vi "System8.vi"() -> ()   [LabVIEW 2015]
uses:
  Control 1.ctl
  <vilib>/DAQmx/write.llb/DAQmx Write (Digital 1D Bool NChan 1Samp 1Line).vi
  <vilib>/DAQmx/write.llb/DAQmx Write (Digital Bool 1Line 1Point).vi
  <vilib>/DAQmx/read.llb/DAQmx Read (Analog DBL 1Chan 1Samp).vi
  <vilib>/DAQmx/read.llb/DAQmx Read (Analog 1D Wfm NChan NSamp).vi
  <vilib>/Analysis/baseanly.llb/Mean (DBL).vi
  <vilib>/DAQmx/write.llb/DAQmx Write (Analog DBL 1Chan 1Samp).vi
  <vilib>/DAQmx/miscellaneous.llb/DAQmx Fill In Error Info.vi
  <vilib>/addons/control/pid/NI_PID_autopid.lvlib
  <vilib>/Analysis/NI_AALBase.lvlib
panel:
  out "Voltage Reading(Temp) 2":dbl format="%#_13g"
  out "Temperature (Celcius) 2":dbl format="%#.1g"
  out "Temp(C) 2":dbl(slide) scale=-10.0..100.0
  out "Temp Chart 3":waveform(dbl)(graph)
  in  "autotuning parameters 4":T1={"controller type"=1, "relay cycles"=3, "relay amplitude"=1.0, "control specification"=2, "PV noise level"=0.1} {"PV noise level" format="%.2f"; "control specification" items=["normal", "fast", "slow"]; "relay amplitude" format="%.2f"; "controller type" items=["PID", "PI", "P"]}
  in  "PID gains 4":T2={"proportional gain (Kc)"=1.0, "integral time (Ti, min)"=0.01, "derivative time (Td, min)"=0.0} {"derivative time (Td, min)" format="%.3f"; "integral time (Ti, min)" format="%.3f"; "proportional gain (Kc)" format="%.3f"}
  out "PID gains out 4":T2={"proportional gain (Kc)"=1.0, "integral time (Ti, min)"=0.01, "derivative time (Td, min)"=0.0} {"derivative time (Td, min)" format="%.3f"; "integral time (Ti, min)" format="%.3f"; "proportional gain (Kc)" format="%.3f"}
  in  "autotune? (F) 4":bool
  in  "reinitialize? (F) 4":bool
  in  "setpoint in C 2":dbl format="%.2f"
  in  "Manual Control 4":bool
  in  "Heater On/Off 2":bool
  out "Voltage Reading(Temp)":dbl format="%#_13g"
  out "Temperature (Celcius)":dbl format="%#.1g"
  out "Temp(C)":dbl(slide) scale=-10.0..100.0
  out "Temp Chart 2":waveform(dbl)(graph)
  in  "autotuning parameters 3":T1={"controller type"=1, "relay cycles"=3, "relay amplitude"=1.0, "control specification"=2, "PV noise level"=0.1} {"PV noise level" format="%.2f"; "control specification" items=["normal", "fast", "slow"]; "relay amplitude" format="%.2f"; "controller type" items=["PID", "PI", "P"]}
  in  "PID gains 3":T2={"proportional gain (Kc)"=1.0, "integral time (Ti, min)"=0.01, "derivative time (Td, min)"=0.0} {"derivative time (Td, min)" format="%.3f"; "integral time (Ti, min)" format="%.3f"; "proportional gain (Kc)" format="%.3f"}
  out "PID gains out 3":T2={"proportional gain (Kc)"=1.0, "integral time (Ti, min)"=0.01, "derivative time (Td, min)"=0.0} {"derivative time (Td, min)" format="%.3f"; "integral time (Ti, min)" format="%.3f"; "proportional gain (Kc)" format="%.3f"}
  in  "autotune? (F) 3":bool
  in  "reinitialize? (F) 3":bool
  in  "setpoint in C":dbl format="%.2f"
  out "Control Value 3":dbl
  in  "Manual Control 3":bool
  in  "Heater On/Off":bool
  in  "Open/Close (Green)":bool
  in  "Open/Close (Blue)":bool
  in  "Stop program":bool
  in  "On/Off":bool
  in  "Manual Control 2":bool
  in  "Voltage setting 2":dbl format="%#_13g"
  out "Voltage Reading(pressure) 2":dbl format="%#_13g"
  out "Pressure 2":dbl format="%#.3g"
  out "Pressure Chart 2":dbl(graph)
  in  "autotuning parameters 2":T1={"controller type"=1, "relay cycles"=3, "relay amplitude"=1.0, "control specification"=2, "PV noise level"=0.1} {"PV noise level" format="%.2f"; "control specification" items=["normal", "fast", "slow"]; "relay amplitude" format="%.2f"; "controller type" items=["PID", "PI", "P"]}
  in  "PID gains 2":T2={"proportional gain (Kc)"=1.0, "integral time (Ti, min)"=0.01, "derivative time (Td, min)"=0.0} {"derivative time (Td, min)" format="%.3f"; "integral time (Ti, min)" format="%.3f"; "proportional gain (Kc)" format="%.3f"}
  out "PID gains out 2":T2={"proportional gain (Kc)"=1.0, "integral time (Ti, min)"=0.01, "derivative time (Td, min)"=0.0} {"derivative time (Td, min)" format="%.3f"; "integral time (Ti, min)" format="%.3f"; "proportional gain (Kc)" format="%.3f"}
  in  "autotune? (F) 2":bool
  in  "reinitialize? (F) 2":bool
  in  "setpoint in Bar 2":dbl format="%#.5f"
  out "Control Value 2":dbl
  in  "Voltage setting":dbl format="%#_13g"
  in  "Manual Control":bool
  out "Control Value":dbl
  in  "setpoint in Bar":dbl format="%#.5f"
  in  "reinitialize? (F)":bool
  in  "autotune? (F)":bool
  out "PID gains out":T2={"proportional gain (Kc)"=1.0, "integral time (Ti, min)"=0.01, "derivative time (Td, min)"=0.0} {"derivative time (Td, min)" format="%.3f"; "integral time (Ti, min)" format="%.3f"; "proportional gain (Kc)" format="%.3f"}
  in  "PID gains":T2={"proportional gain (Kc)"=1.0, "integral time (Ti, min)"=0.01, "derivative time (Td, min)"=0.0} {"derivative time (Td, min)" format="%.3f"; "integral time (Ti, min)" format="%.3f"; "proportional gain (Kc)" format="%.3f"}
  in  "autotuning parameters":T1={"controller type"=1, "relay cycles"=3, "relay amplitude"=1.0, "control specification"=2, "PV noise level"=0.1} {"PV noise level" format="%.2f"; "control specification" items=["normal", "fast", "slow"]; "relay amplitude" format="%.2f"; "controller type" items=["PID", "PI", "P"]}
  out "Pressure Chart":dbl(graph)
  out "Pressure":dbl format="%#.3g"
  out "Voltage Reading(pressure)":dbl format="%#_13g"
  # "Valves"
  # "Pump 3"
  # "Pressure Vessel 2"
  # "Pressure Vessel 1"
  # "Readings"
  # "Controls"
  # "Readings"
  # "Controls"
  # "PID Settings"
  # "51.12139\n\n0.044676"
  # "Temperature 1"
  # "Temperature 2"
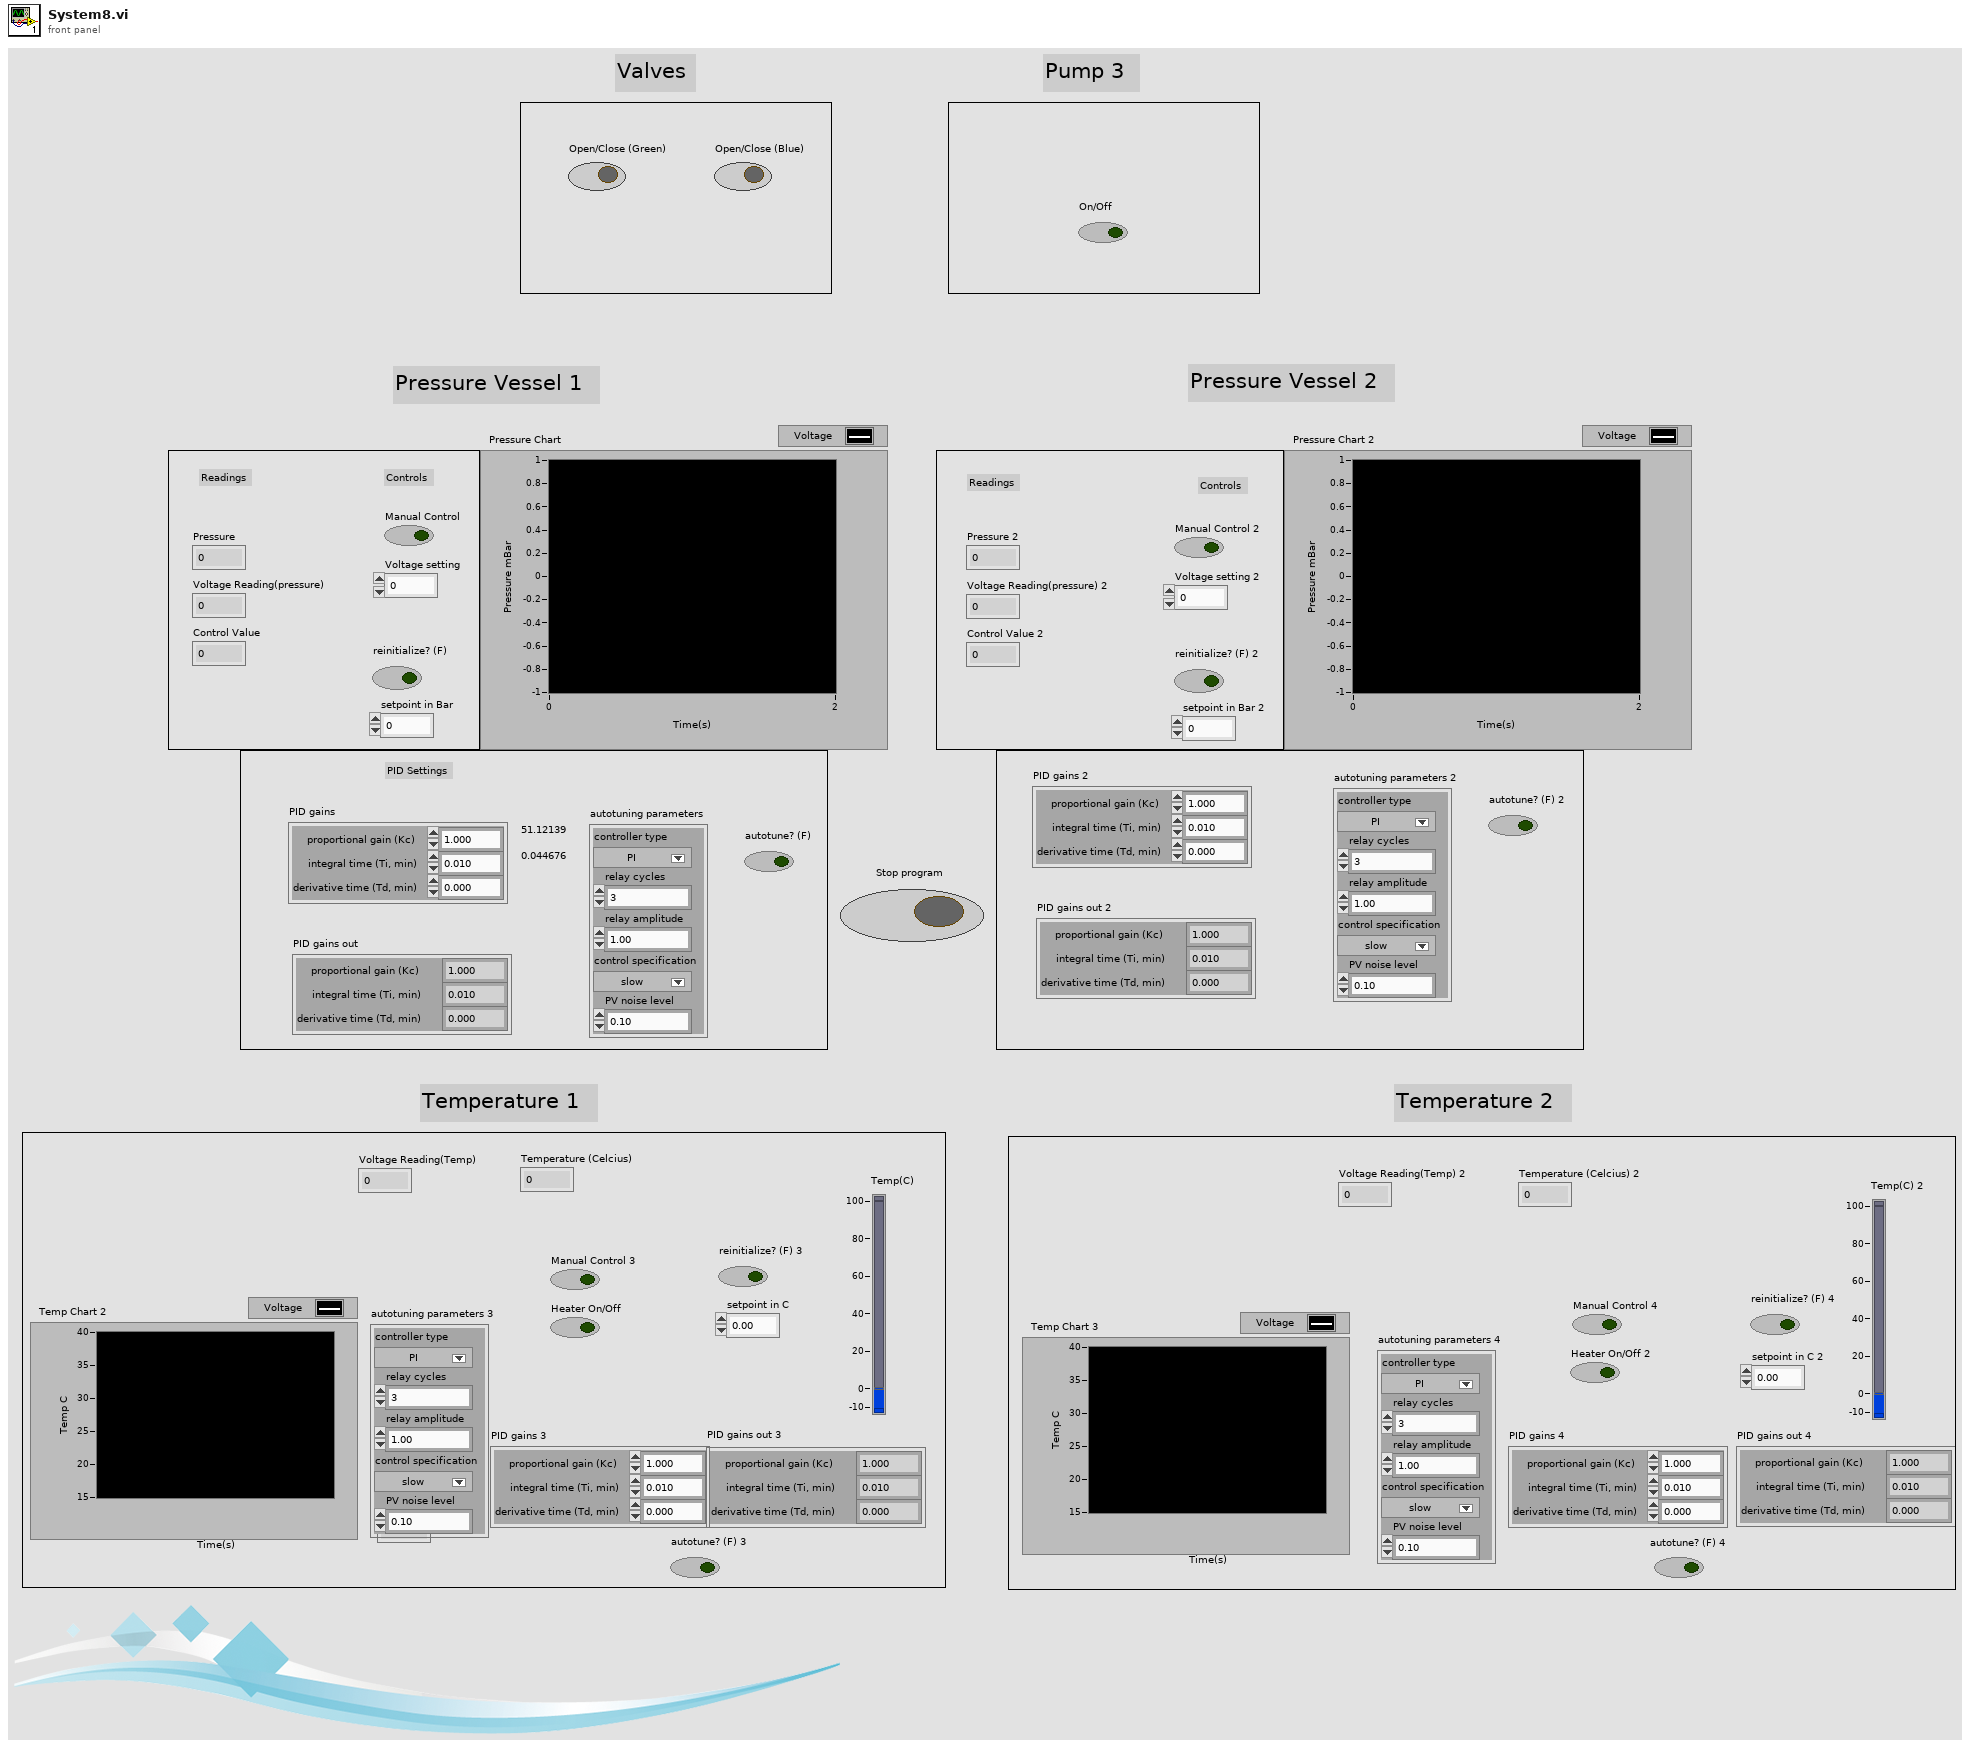
[diagram p1: front panel]
types:
  T1 = cluster{"controller type":u16, "relay cycles":i32, "relay amplitude":dbl, "control specification":u16, "PV noise level":dbl}
  T2 = cluster{"proportional gain (Kc)":dbl, "integral time (Ti, min)":dbl, "derivative time (Td, min)":dbl}
  T3 = typedef "Control 1.ctl" = refnum<k21>
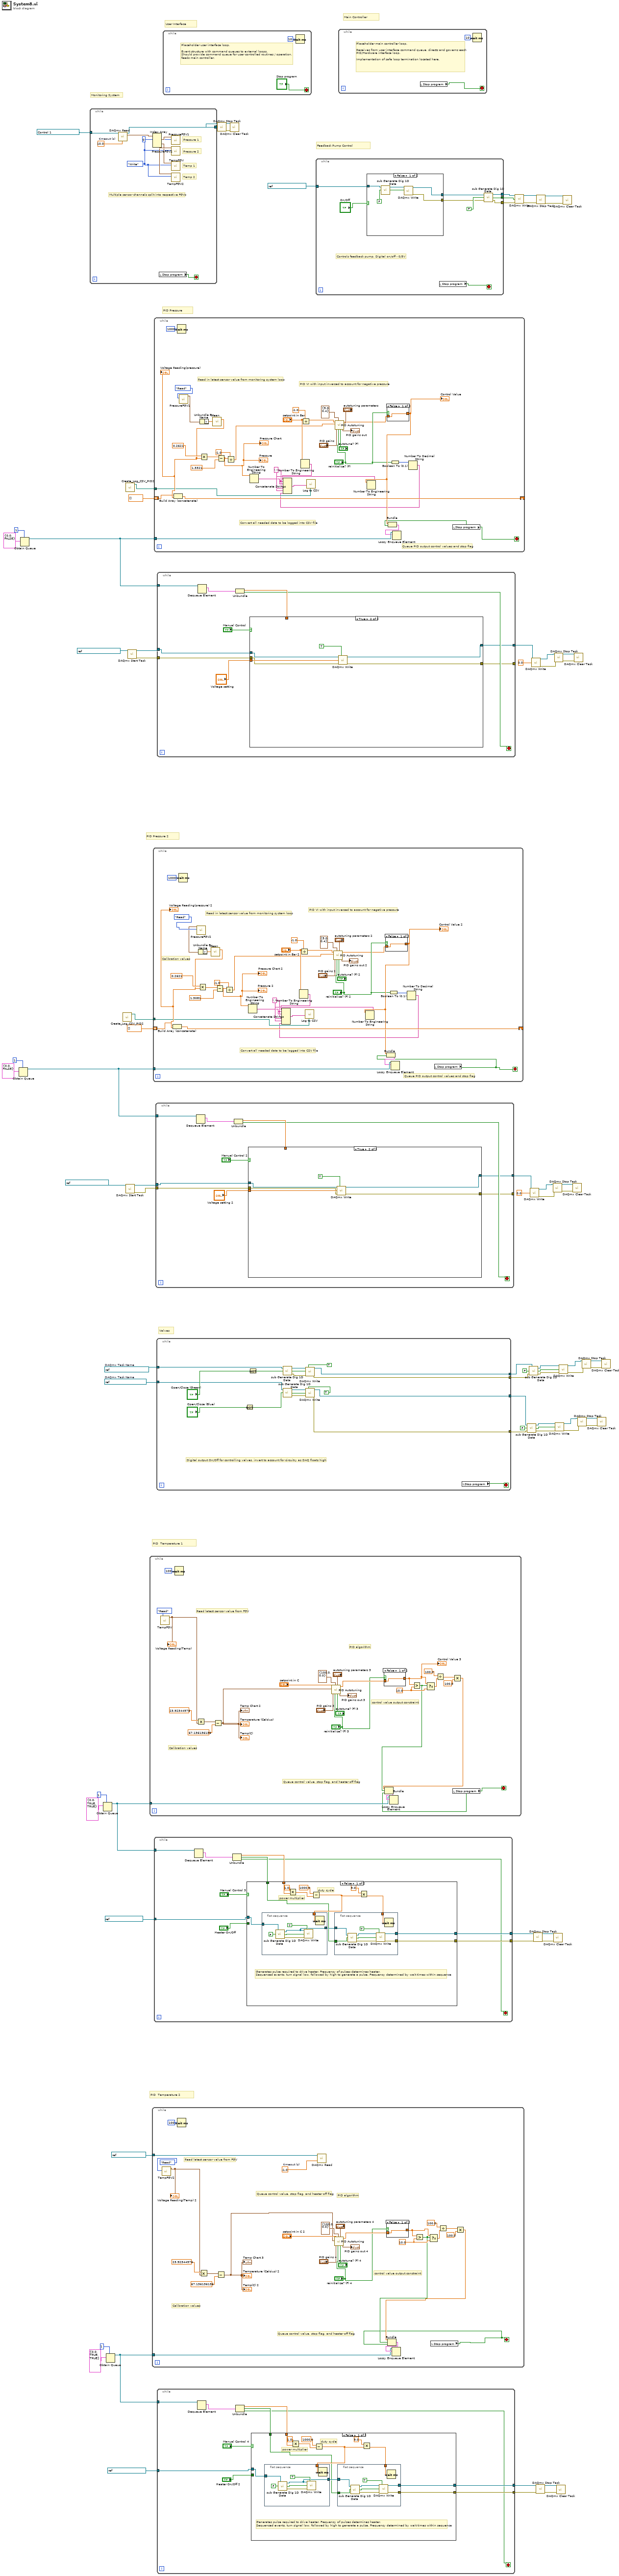
[diagram p0: block diagram]
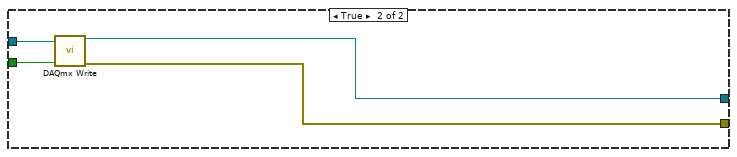
[diagram p2: hidden frame]
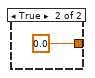
[diagram p3: hidden frame]
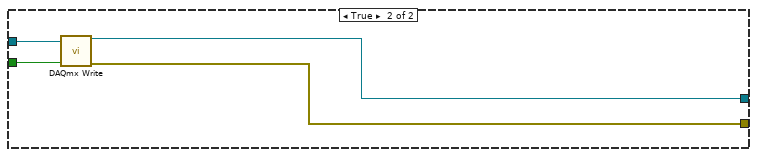
[diagram p4: hidden frame]
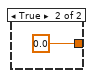
[diagram p5: hidden frame]
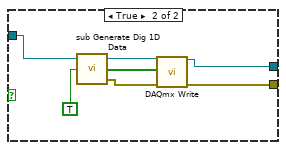
[diagram p6: hidden frame]
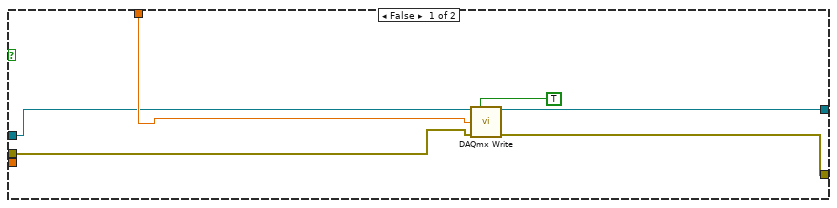
[diagram p7: hidden frame]
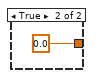
[diagram p8: hidden frame]
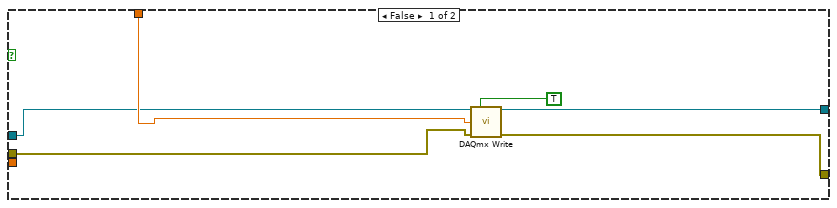
[diagram p9: hidden frame]
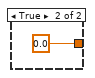
[diagram p10: hidden frame]
diagram:
  w45 = refnum<k21> "NewDigitalSystemBlue"  # DAQmx Task Name
  w46 = refnum<k21> "NewDigitalSystemGreen"  # DAQmx Task Name
  # "Main Controller"
  # "User Interface"
  # "Feedback Pump Control"
  # "PID  Temperature 2"
  # "PID  Temperature 1"
  # "Monitoring System"
  # "Valves"
  # "PID Pressure"
  # "PID Pressure 2"
  n1 = Obtain Queue(max queue size (-1, unlimited)=1, element data type=cluster{dbl, bool} {0.0, FALSE}) -> (queue out=w64:refnum<queue>)  [unwired: 3 in, 2 out]
  n2 = Obtain Queue(max queue size (-1, unlimited)=1, element data type=cluster{dbl, bool} {0.0, FALSE}) -> (queue out=w78:refnum<queue>)  [unwired: 3 in, 2 out]
  n3 = while {
    tunnel: T3 "New AnalogSystemAI0" -> [w88]
    tunnel: [w87] -> w21
    stop <- w90 stop-if-true
    w80 = enum16{"Write", "Read"}."Write" ("Command")
    w89 = 10.0  # timeout (s)
    # "Multiple sensor channels split into respective FGVs"
    # "Temp 2"
    # "Temp 1"
    # "Pressure 2"
    # "Pressure 1"
    n4 = call-poly <vilib>:"DAQmx Read.vi"("task/channels in"=w88, "timeout"=w89) -> ("task out"=w87:refnum<k21>, "data"=w85:waveform(dbl)[])  [unwired: 11 in, 1 out]
    n5 = Index Array(array=w85, index #1=0 ("index")) -> (element #1=w84:waveform(dbl), element #2=w83:waveform(dbl), element #3=w82:waveform(dbl), element #4=w81:waveform(dbl))  [unwired: 3 in]
    n6 = local read "Stop program"() -> (w90:bool)
    n7 = call "PressureFGV1.vi"("Command"=w80, "element"=w84) -> ()  [unwired: 9 in, 1 out]
    n8 = call "PressureFGV2.vi"("Command"=w80, "element"=w83) -> ()  [unwired: 9 in, 1 out]
    n9 = call "TempFGV.vi"("Command"=w80, "element 3"=w82) -> ()  [unwired: 9 in, 1 out]
    n10 = call "TempFGV2.vi"("Command"=w80, "element 3"=w81) -> ()  [unwired: 9 in, 1 out]
  }
  n11 = Obtain Queue(max queue size (-1, unlimited)=1, element data type=cluster{dbl, bool, bool} {0.0, TRUE, TRUE}) -> (queue out=w14:refnum<queue>)  [unwired: 3 in, 2 out]
  n12 = Obtain Queue(max queue size (-1, unlimited)=1, element data type=cluster{dbl, bool, bool} {0.0, TRUE, TRUE}) -> (queue out=w10:refnum<queue>)  [unwired: 3 in, 2 out]
  n13 = call "Create_Log_CSV_PID2.vi"() -> ("path"=w60:path)  [unwired: 11 in]
  n14 = call "Create_Log_CSV_PID2.vi"() -> ("path"=w74:path)  [unwired: 11 in]
  n15 = call <vilib>:"DAQmx Start Task.vi"("task/channels in"=refnum<k21> "NewAnalogSystemAO1") -> ("task out"=w59:refnum<k21>, "error out"=w58:errorcluster)  [unwired: 13 in]
  n16 = call <vilib>:"DAQmx Start Task.vi"("task/channels in"=refnum<k21> "NewAnalogSystemAO0") -> ("task out"=w73:refnum<k21>, "error out"=w72:errorcluster)  [unwired: 13 in]
  n17 = while {
    tunnel: w14 -> [w94]
    stop <- w93 stop-if-true
    w100 = 10.0 ("f")
    # "Queue control value, stop flag, and heater off flag"
    # "Calibration values"
    # "control value output constraint"
    # "PID algorithm"
    # "Read latest sensor value from FGV"
    n18 = call "TempFGV.vi"("Command"=enum16{"Write", "Read"}."Read") -> ("element 2"=w91:waveform(dbl))  [unwired: 10 in]
    "Voltage Reading(Temp)" <- w91
    n19 = Wait (ms)(milliseconds to wait=u32 100) -> ()  [unwired: 1 out]
    n20 = Multiply(x=23.92344976, y=w91) -> (x*y=w115:waveform(dbl))
    n21 = Subtract(x=w115, y=67.136136136) -> (x-y=w98:waveform(dbl))
    "Temperature (Celcius)" <- w98
    "Temp(C)" <- w98
    "Temp Chart 2" <- w98
    n22 = call <vilib>:"PID Autotuning.vi"("autotune? (F)"="autotune? (F) 3", "autotuning parameters"="autotuning parameters 3", "reinitialize? (F)"="reinitialize? (F) 3", "output range"=cluster{"output high":dbl, "output low":dbl} {"output high"=100.0, "output low"=0.0}, "PID gains"="PID gains 3", "process variable"=w98, "setpoint"="setpoint in C") -> ("PID gains out"=→"PID gains out 3":T2, "output"=w108:dbl)  [unwired: 1 in, 2 out]
    n23 = case shown="False" "reinitialize? (F) 3" {
      tunnel: [w117 0.0] -> w101
      tunnel: w108 -> [w117 _]
      frame False {
      }
      frame True {
      }
    }
    "Control Value 3" <- w101
    n24 = Greater?(x=w101, y=w100) -> (0:w96:bool)
    n25 = Select(t=w101, s=w96, f=w100) -> (s? t:f=w102:dbl)
    n26 = Divide(x=100.0, y=w102) -> (x/y=w104:dbl)
    n27 = local read "Stop program"() -> (w93:bool)
    n28 = Multiply(x=w104, y=100.0) -> (x*y=w97:dbl)
    n29 = Bundle(w97, w96, "Stop program"=w93) -> (w95:cluster{dbl, bool, "Stop program":bool})  [unwired: 1 in]
    n30 = Lossy Enqueue Element(queue=w94, element=w95) -> ()  [unwired: 1 in, 4 out]
  }
  n31 = while {
    tunnel: refnum<k21> "MyVoltageTask_0" -> [w142]
    tunnel: w10 -> [w122]
    stop <- w119 stop-if-true
    w128 = 10.0 ("f")
    w146 = -1.0  # timeout (s)
    # "Queue control value, stop flag, and heater off flag"
    # "Queue control value, stop flag, and heater off flag"
    # "Calibration values"
    # "control value output constraint"
    # "PID algorithm"
    # "Read latest sensor value from FGV"
    n32 = call "TempFGV2.vi"("Command"=enum16{"Write", "Read"}."Read") -> ("element 2"=w120:waveform(dbl))  [unwired: 10 in]
    "Voltage Reading(Temp) 2" <- w120
    n33 = Wait (ms)(milliseconds to wait=u32 100) -> ()  [unwired: 1 out]
    n34 = Multiply(x=23.92344976, y=w120) -> (x*y=w144:waveform(dbl))
    n35 = Subtract(x=w144, y=67.136136136) -> (x-y=w126:waveform(dbl))
    "Temperature (Celcius) 2" <- w126
    "Temp(C) 2" <- w126
    "Temp Chart 3" <- w126
    n36 = call-poly <vilib>:"DAQmx Read.vi"("task/channels in"=w142, "timeout"=w146) -> ()  [unwired: 11 in, 3 out]
    n37 = call <vilib>:"PID Autotuning.vi"("autotune? (F)"="autotune? (F) 4", "autotuning parameters"="autotuning parameters 4", "reinitialize? (F)"="reinitialize? (F) 4", "output range"=cluster{"output high":dbl, "output low":dbl} {"output high"=100.0, "output low"=0.0}, "PID gains"="PID gains 4", "process variable"=w126, "setpoint"="setpoint in C 2") -> ("PID gains out"=→"PID gains out 4":T2, "output"=w136:dbl)  [unwired: 1 in, 2 out]
    n38 = case shown="False" "reinitialize? (F) 4" {
      tunnel: [w147 0.0] -> w129
      tunnel: w136 -> [w147 _]
      frame False {
      }
      frame True {
      }
    }
    n39 = Greater?(x=w129, y=w128) -> (0:w124:bool)
    n40 = Select(t=w129, s=w124, f=w128) -> (s? t:f=w130:dbl)
    n41 = local read "Stop program"() -> (w119:bool)
    n42 = Divide(x=100.0, y=w130) -> (x/y=w132:dbl)
    n43 = Multiply(x=w132, y=100.0) -> (x*y=w125:dbl)
    n44 = Bundle(w125, w124, "Stop program"=w119) -> (w123:cluster{dbl, bool, "Stop program":bool})  [unwired: 1 in]
    n45 = Lossy Enqueue Element(queue=w122, element=w123) -> ()  [unwired: 1 in, 4 out]
  }
  n46 = while {
    tunnel: w64 -> [w175]
    shift-right: [w172] -> _
    shift-left: dbl[] [] -> [w173]
    tunnel: w60 -> [w166]
    stop <- w153 stop-if-true
    w161 = ","
    # "Calibration values"
    # "Queue PID output control values and stop flag"
    # "Convert all needed data to be logged into CSV file"
    # "PID VI with input inversed to account for negative pressure"
    # "Read in latest sensor value from monitoring system loop"
    n47 = Wait (ms)(milliseconds to wait=u32 1000) -> ()  [unwired: 1 out]
    n48 = call "PressureFGV2.vi"("Command"=enum16{"Write", "Read"}."Read") -> ("element 2"=w149:waveform(dbl))  [unwired: 10 in]
    n49 = Unbundle By Name(w149) -> ("Y"=w151:dbl[])
    n50 = call-poly <vilib>:"Mean.vi"("X"=w151) -> ("mean"=w174:dbl)  [unwired: 1 out]
    "Voltage Reading(pressure) 2" <- w174
    n51 = Build Array (concatenate)(w173, w174) -> (w172:dbl[])
    n52 = Multiply(x=0.2621, y=w174) -> (x*y=w182:dbl)
    n53 = Subtract(x=w182, y=1.3081) -> (x-y=w170:dbl)
    "Pressure 2" <- w170
    "Pressure Chart 2" <- w170
    n54 = Divide(x=w170, y=-1.0) -> (x/y=w158:dbl)
    n55 = Number To Engineering String(4:w170) -> (0:w165:string)  [unwired: 3 in]
    n56 = Number To Engineering String(4:"setpoint in Bar 2") -> (0:w164:string)  [unwired: 3 in]
    n57 = Divide(x="setpoint in Bar 2", y=-1.0) -> (x/y=w157:dbl)
    n58 = call <vilib>:"PID Autotuning.vi"("autotune? (F)"="autotune? (F) 2", "autotuning parameters"="autotuning parameters 2", "reinitialize? (F)"="reinitialize? (F) 2", "output range"=cluster{"output high":dbl, "output low":dbl} {"output high"=5.0, "output low"=0.4}, "PID gains"="PID gains 2", "process variable"=w158, "setpoint"=w157) -> ("PID gains out"=→"PID gains out 2":T2, "output"=w155:dbl)  [unwired: 1 in, 2 out]
    n59 = case shown="False" "reinitialize? (F) 2" {
      tunnel: [w184 0.0] -> w169
      tunnel: w155 -> [w184 _]
      frame False {
      }
      frame True {
      }
    }
    "Control Value 2" <- w169
    n60 = Number To Engineering String(4:w169) -> (0:w168:string)  [unwired: 3 in]
    n61 = Boolean To (0,1)(Boolean="reinitialize? (F) 2") -> (0, 1=w162:i16)
    n62 = Number To Decimal String(number=w162) -> (decimal integer string=w160:string)  [unwired: 1 in]
    n63 = Concatenate Strings(w164, w161, w165, w161, w168, w161, w160) -> (w167:string)
    n64 = call "Log to CSV.vi"("Data Str"=w167, "Path"=w166) -> ()  [unwired: 5 in, 1 out]
    n65 = local read "Stop program"() -> (w153:bool)
    n66 = Bundle("output"=w169, "Stop program"=w153) -> (w154:cluster{"output":dbl, "Stop program":bool})  [unwired: 1 in]
    n67 = Lossy Enqueue Element(queue=w175, element=w154) -> ()  [unwired: 1 in, 4 out]
  }
  n68 = while {
    tunnel: w14 -> [w195]
    tunnel: refnum<k21> "MyDigitalOutTask_2" -> [w192]
    tunnel: [w188] -> w17
    tunnel: [w187] -> w18
    stop <- w186 stop-if-true
    n69 = Dequeue Element(queue=w195) -> (element=w191:cluster{dbl, bool, bool})  [unwired: 2 in, 3 out]
    n70 = Unbundle(w191) -> (w190:dbl, w189:bool, w186:bool)
    n71 = case shown="False" "Manual Control 3" {
      tunnel: w192 -> [w206 w227]
      tunnel: "Heater On/Off" -> [_ w226]
      tunnel: w190 -> [w205 _]
      tunnel: w189 -> [w200 _]
      tunnel: [w197 w225] -> w188
      tunnel: [w196 w224] -> w187
      frame False {
        # "Generates pulse required to drive heater. Frequency of pulses determines heater.\nSequenced events, turn signal low, followed by high to generate a pulse. Frequency determined by wait times within sequence"
        # "duty cycle"
        # "power multiplier"
        n72 = flat-sequence {
          tunnel: w206 -> [w220]
          tunnel: [w219] -> w207
          tunnel: w204 -> [w218]
          frame #0 {
            n73 = call <vilib>:"sub Generate Dig 1D Data.vi"("initial value"=FALSE, "task in"=w220) -> ("error out"=w222:errorcluster, "Data"=w223:bool[], "task out"=w219:refnum<k21>)  [unwired: 1 in]
            n74 = call-poly <vilib>:"DAQmx Write.vi"("task/channels in"=w219, "auto start"=TRUE, "data"=w223, "error in"=w222) -> ()  [unwired: 9 in, 3 out]
            n75 = Wait (ms)(milliseconds to wait=w218) -> ()  [unwired: 1 out]
          }
        }
        n76 = Multiply(x=1.0, y=w205) -> (x*y=w199:dbl)
        n77 = Subtract(x=1000.0, y=w199) -> (x-y=w204:dbl)
        n78 = flat-sequence {
          tunnel: w207 -> [w212]
          tunnel: w202 -> [w211]
          tunnel: w200 -> [w210]
          tunnel: [w209] -> w197
          tunnel: [w208] -> w196
          frame #0 {
            n79 = call <vilib>:"sub Generate Dig 1D Data.vi"("initial value"=w210, "task in"=w212) -> ("error out"=w215:errorcluster, "Data"=w213:bool[], "task out"=w214:refnum<k21>)  [unwired: 1 in]
            n80 = call-poly <vilib>:"DAQmx Write.vi"("task/channels in"=w214, "auto start"=TRUE, "data"=w213, "error in"=w215) -> ("task out"=w209:refnum<k21>, "error out"=w208:errorcluster)  [unwired: 9 in, 1 out]
            n81 = Wait (ms)(milliseconds to wait=w211) -> ()  [unwired: 1 out]
          }
        }
        n82 = Multiply(x=9.0, y=w204) -> (x*y=w202:dbl)
      }
      frame True {
        n83 = call-poly <vilib>:"DAQmx Write.vi"("task/channels in"=w227, "data"=w226) -> ("task out"=w225:refnum<k21>, "error out"=w224:errorcluster)  [unwired: 11 in, 1 out]
      }
    }
  }
  n84 = while {
    tunnel: w78 -> [w254]
    shift-right: [w249] -> _
    shift-left: dbl[] [] -> [w250]
    tunnel: w74 -> [w243]
    stop <- w231 stop-if-true
    w238 = ","
    # "Queue PID output control values and stop flag"
    # "Convert all needed data to be logged into CSV file"
    # "PID VI with input inversed to account for negative pressure"
    # "Read in latest sensor value from monitoring system loop"
    n85 = Wait (ms)(milliseconds to wait=u32 1000) -> ()  [unwired: 1 out]
    n86 = call "PressureFGV1.vi"("Command"=enum16{"Write", "Read"}."Read") -> ("element 2"=w228:waveform(dbl))  [unwired: 10 in]
    n87 = Unbundle By Name(w228) -> ("Y"=w252:dbl[])
    n88 = call-poly <vilib>:"Mean.vi"("X"=w252) -> ("mean"=w251:dbl)  [unwired: 1 out]
    "Voltage Reading(pressure)" <- w251
    n89 = Build Array (concatenate)(w250, w251) -> (w249:dbl[])
    n90 = Multiply(x=0.2621, y=w251) -> (x*y=w261:dbl)
    n91 = Subtract(x=w261, y=1.3321) -> (x-y=w247:dbl)
    "Pressure" <- w247
    "Pressure Chart" <- w247
    n92 = Divide(x=w247, y=-1.0) -> (x/y=w235:dbl)
    n93 = Number To Engineering String(4:w247) -> (0:w242:string)  [unwired: 3 in]
    n94 = Number To Engineering String(4:"setpoint in Bar") -> (0:w241:string)  [unwired: 3 in]
    n95 = Divide(x="setpoint in Bar", y=-1.0) -> (x/y=w234:dbl)
    n96 = call <vilib>:"PID Autotuning.vi"("autotune? (F)"="autotune? (F)", "autotuning parameters"="autotuning parameters", "reinitialize? (F)"="reinitialize? (F)", "output range"=cluster{"output high":dbl, "output low":dbl} {"output high"=5.0, "output low"=0.4}, "PID gains"="PID gains", "process variable"=w235, "setpoint"=w234) -> ("PID gains out"=→"PID gains out":T2, "output"=w232:dbl)  [unwired: 1 in, 2 out]
    n97 = case shown="False" "reinitialize? (F)" {
      tunnel: [w263 0.0] -> w246
      tunnel: w232 -> [w263 _]
      frame False {
      }
      frame True {
      }
    }
    "Control Value" <- w246
    n98 = Number To Engineering String(4:w246) -> (0:w245:string)  [unwired: 3 in]
    n99 = Boolean To (0,1)(Boolean="reinitialize? (F)") -> (0, 1=w239:i16)
    n100 = Number To Decimal String(number=w239) -> (decimal integer string=w237:string)  [unwired: 1 in]
    n101 = Concatenate Strings(w241, w238, w242, w238, w245, w238, w237) -> (w244:string)
    n102 = call "Log to CSV.vi"("Data Str"=w244, "Path"=w243) -> ()  [unwired: 5 in, 1 out]
    n103 = local read "Stop program"() -> (w231:bool)
    n104 = Bundle("output"=w246, "Stop program"=w231) -> (w253:cluster{"output":dbl, "Stop program":bool})  [unwired: 1 in]
    n105 = Lossy Enqueue Element(queue=w254, element=w253) -> ()  [unwired: 1 in, 4 out]
  }
  n106 = while {
    tunnel: w64 -> [w274]
    tunnel: w59 -> [w272]
    tunnel: [w267] -> w56
    tunnel: w58 -> [w266]
    tunnel: [w265] -> _
    stop <- w268 stop-if-true
    n107 = Dequeue Element(queue=w274) -> (element=w271:cluster{dbl, bool})  [unwired: 2 in, 3 out]
    n108 = Unbundle(w271) -> (w270:dbl, w268:bool)
    n109 = case shown="True" "Manual Control 2" {
      tunnel: w272 -> [w278 w285]
      tunnel: w270 -> [w279 _]
      tunnel: "Voltage setting 2" -> [_ w284]
      tunnel: [w277 w283] -> w267
      tunnel: w266 -> [w276 w282]
      tunnel: [w275 w281] -> w265
      frame False {
        n110 = call-poly <vilib>:"DAQmx Write.vi"("task/channels in"=w278, "auto start"=TRUE, "data"=w279, "error in"=w276) -> ("task out"=w277:refnum<k21>, "error out"=w275:errorcluster)  [unwired: 9 in, 1 out]
      }
      frame True {
        n111 = call-poly <vilib>:"DAQmx Write.vi"("task/channels in"=w285, "auto start"=TRUE, "data"=w284, "error in"=w282) -> ("task out"=w283:refnum<k21>, "error out"=w281:errorcluster)  [unwired: 9 in, 1 out]
      }
    }
  }
  n112 = while {
    tunnel: w46 -> [w295]
    tunnel: w45 -> [w294]
    tunnel: [w293] -> w35
    tunnel: [w292] -> w31
    tunnel: [w289] -> w28
    tunnel: [w288] -> w26
    stop <- w287 stop-if-true
    # "Digital output On/Off for controlling valves, invert to account for circuitry as DAQ floats high"
    n113 = Not(x="Open/Close (Blue)") -> (.not. x?=w305:bool)
    n114 = Not(x="Open/Close (Green)") -> (.not. x?=w304:bool)
    n115 = call <vilib>:"sub Generate Dig 1D Data.vi"("initial value"=w304, "task in"=w295) -> ("error out"=w291:errorcluster, "Data"=w302:bool[], "task out"=w299:refnum<k21>)  [unwired: 1 in]
    n116 = call <vilib>:"sub Generate Dig 1D Data.vi"("initial value"=w305, "task in"=w294) -> ("error out"=w290:errorcluster, "Data"=w301:bool[], "task out"=w300:refnum<k21>)  [unwired: 1 in]
    n117 = call-poly <vilib>:"DAQmx Write.vi"("task/channels in"=w299, "auto start"=TRUE, "data"=w302, "error in"=w291) -> ("task out"=w293:refnum<k21>, "error out"=w289:errorcluster)  [unwired: 9 in, 1 out]
    n118 = call-poly <vilib>:"DAQmx Write.vi"("task/channels in"=w300, "auto start"=TRUE, "data"=w301, "error in"=w290) -> ("task out"=w292:refnum<k21>, "error out"=w288:errorcluster)  [unwired: 9 in, 1 out]
    n119 = local read "Stop program"() -> (w287:bool)
  }
  n120 = while {
    tunnel: w10 -> [w315]
    tunnel: refnum<k21> "MyDigitalOutTask_2" -> [w312]
    tunnel: [w308] -> w7
    tunnel: [w307] -> w6
    stop <- w306 stop-if-true
    n121 = Dequeue Element(queue=w315) -> (element=w311:cluster{dbl, bool, bool})  [unwired: 2 in, 3 out]
    n122 = Unbundle(w311) -> (w310:dbl, w309:bool, w306:bool)
    n123 = case shown="False" "Manual Control 4" {
      tunnel: w312 -> [w326 w347]
      tunnel: "Heater On/Off 2" -> [_ w346]
      tunnel: w310 -> [w325 _]
      tunnel: w309 -> [w320 _]
      tunnel: [w317 w345] -> w308
      tunnel: [w316 w344] -> w307
      frame False {
        # "Generates pulse required to drive heater. Frequency of pulses determines heater.\nSequenced events, turn signal low, followed by high to generate a pulse. Frequency determined by wait times within sequence"
        # "duty cycle"
        # "power multiplier"
        n124 = flat-sequence {
          tunnel: w326 -> [w340]
          tunnel: [w339] -> w327
          tunnel: w324 -> [w338]
          frame #0 {
            n125 = call <vilib>:"sub Generate Dig 1D Data.vi"("initial value"=FALSE, "task in"=w340) -> ("error out"=w342:errorcluster, "Data"=w343:bool[], "task out"=w339:refnum<k21>)  [unwired: 1 in]
            n126 = call-poly <vilib>:"DAQmx Write.vi"("task/channels in"=w339, "auto start"=TRUE, "data"=w343, "error in"=w342) -> ()  [unwired: 9 in, 3 out]
            n127 = Wait (ms)(milliseconds to wait=w338) -> ()  [unwired: 1 out]
          }
        }
        n128 = Multiply(x=1.0, y=w325) -> (x*y=w319:dbl)
        n129 = Subtract(x=1000.0, y=w319) -> (x-y=w324:dbl)
        n130 = flat-sequence {
          tunnel: w327 -> [w332]
          tunnel: w322 -> [w331]
          tunnel: w320 -> [w330]
          tunnel: [w329] -> w317
          tunnel: [w328] -> w316
          frame #0 {
            n131 = call <vilib>:"sub Generate Dig 1D Data.vi"("initial value"=w330, "task in"=w332) -> ("error out"=w335:errorcluster, "Data"=w333:bool[], "task out"=w334:refnum<k21>)  [unwired: 1 in]
            n132 = call-poly <vilib>:"DAQmx Write.vi"("task/channels in"=w334, "auto start"=TRUE, "data"=w333, "error in"=w335) -> ("task out"=w329:refnum<k21>, "error out"=w328:errorcluster)  [unwired: 9 in, 1 out]
            n133 = Wait (ms)(milliseconds to wait=w331) -> ()  [unwired: 1 out]
          }
        }
        n134 = Multiply(x=9.0, y=w324) -> (x*y=w322:dbl)
      }
      frame True {
        n135 = call-poly <vilib>:"DAQmx Write.vi"("task/channels in"=w347, "data"=w346) -> ("task out"=w345:refnum<k21>, "error out"=w344:errorcluster)  [unwired: 11 in, 1 out]
      }
    }
  }
  n136 = while {
    tunnel: w78 -> [w357]
    tunnel: w73 -> [w355]
    tunnel: [w350] -> w70
    tunnel: w72 -> [w349]
    tunnel: [w348] -> _
    stop <- w351 stop-if-true
    n137 = Dequeue Element(queue=w357) -> (element=w354:cluster{dbl, bool})  [unwired: 2 in, 3 out]
    n138 = Unbundle(w354) -> (w353:dbl, w351:bool)
    n139 = case shown="True" "Manual Control" {
      tunnel: w355 -> [w361 w368]
      tunnel: w353 -> [w362 _]
      tunnel: "Voltage setting" -> [_ w367]
      tunnel: [w360 w366] -> w350
      tunnel: w349 -> [w359 w365]
      tunnel: [w358 w364] -> w348
      frame False {
        n140 = call-poly <vilib>:"DAQmx Write.vi"("task/channels in"=w361, "auto start"=TRUE, "data"=w362, "error in"=w359) -> ("task out"=w360:refnum<k21>, "error out"=w358:errorcluster)  [unwired: 9 in, 1 out]
      }
      frame True {
        n141 = call-poly <vilib>:"DAQmx Write.vi"("task/channels in"=w368, "auto start"=TRUE, "data"=w367, "error in"=w365) -> ("task out"=w366:refnum<k21>, "error out"=w364:errorcluster)  [unwired: 9 in, 1 out]
      }
    }
  }
  n142 = while {
    stop <- "Stop program" stop-if-true
    # "Placeholder user interface loop.\n\nEvent structure with command queues to external loops.\nShould provide command queue for user controlled routines / operation,  \nfeeds main controller."
    n143 = Wait (ms)(milliseconds to wait=u32 10) -> ()  [unwired: 1 out]
  }
  n144 = call <vilib>:"DAQmx Stop Task.vi"("task/channels in"=w21) -> ("task out"=w23:refnum<k21>, "error out"=w22:errorcluster)  [unwired: 13 in]
  n145 = call <vilib>:"DAQmx Clear Task.vi"("task in"=w23, "error in"=w22) -> ()  [unwired: 13 in, 1 out]
  n146 = while {
    tunnel: refnum<k21> "NewDigSystemP0L2" -> [w379]
    tunnel: [w374] -> w3
    tunnel: [w373] -> w2
    tunnel: [w372] -> w1
    stop <- w378 stop-if-true
    # "Controls feedback pump, Digital on/off - 0/5V"
    n147 = case shown="False" "On/Off" {
      tunnel: w379 -> [w386 w390]
      tunnel: [w382 w389] -> w376
      tunnel: [w381 w387] -> w375
      frame False {
        n148 = call <vilib>:"sub Generate Dig 1D Data.vi"("initial value"=FALSE, "task in"=w386) -> ("Data"=w384:bool[], "task out"=w385:refnum<k21>)  [unwired: 1 in, 1 out]
        n149 = call-poly <vilib>:"DAQmx Write.vi"("task/channels in"=w385, "data"=w384) -> ("task out"=w382:refnum<k21>, "error out"=w381:errorcluster)  [unwired: 11 in, 1 out]
      }
      frame True {
        n150 = call <vilib>:"sub Generate Dig 1D Data.vi"("initial value"=TRUE, "task in"=w390) -> ("error out"=w388:errorcluster, "Data"=w392:bool[], "task out"=w391:refnum<k21>)  [unwired: 1 in]
        n151 = call-poly <vilib>:"DAQmx Write.vi"("task/channels in"=w391, "data"=w392, "error in"=w388) -> ("task out"=w389:refnum<k21>, "error out"=w387:errorcluster)  [unwired: 10 in, 1 out]
      }
    }
    n152 = local read "Stop program"() -> (w378:bool)
    n153 = call <vilib>:"sub Generate Dig 1D Data.vi"("error in"=w375, "initial value"=FALSE, "task in"=w376) -> ("error out"=w374:errorcluster, "Data"=w373:bool[], "task out"=w372:refnum<k21>)
  }
  n154 = while {
    stop <- w395 stop-if-true
    # "Placeholder main controller loop.\n\nReceives from user interface command queue, directs and governs each\nPID/Hardware interface loop.\n\nImplementation of safe loop termination located here."
    n155 = local read "Stop program"() -> (w395:bool)
    n156 = Wait (ms)(milliseconds to wait=u32 10) -> ()  [unwired: 1 out]
  }
  n157 = call-poly <vilib>:"DAQmx Write.vi"("task/channels in"=w1, "data"=w2, "error in"=w3) -> ("task out"=w48:refnum<k21>, "error out"=w47:errorcluster)  [unwired: 10 in, 1 out]
  n158 = call <vilib>:"sub Generate Dig 1D Data.vi"("error in"=w26, "initial value"=FALSE, "task in"=w31) -> ("error out"=w25:errorcluster, "Data"=w30:bool[], "task out"=w32:refnum<k21>)
  n159 = call <vilib>:"sub Generate Dig 1D Data.vi"("error in"=w28, "initial value"=FALSE, "task in"=w35) -> ("error out"=w27:errorcluster, "Data"=w29:bool[], "task out"=w36:refnum<k21>)
  n160 = call-poly <vilib>:"DAQmx Write.vi"("task/channels in"=w56, "data"=0.0) -> ("task out"=w55:refnum<k21>, "error out"=w54:errorcluster)  [unwired: 11 in, 1 out]
  n161 = call-poly <vilib>:"DAQmx Write.vi"("task/channels in"=w70, "data"=0.0) -> ("task out"=w69:refnum<k21>, "error out"=w68:errorcluster)  [unwired: 11 in, 1 out]
  n162 = call <vilib>:"DAQmx Stop Task.vi"("task/channels in"=w17, "error in"=w18) -> ("task out"=w19:refnum<k21>, "error out"=w20:errorcluster)  [unwired: 12 in]
  n163 = call <vilib>:"DAQmx Stop Task.vi"("task/channels in"=w7, "error in"=w6) -> ("task out"=w5:refnum<k21>, "error out"=w4:errorcluster)  [unwired: 12 in]
  n164 = call <vilib>:"DAQmx Stop Task.vi"("task/channels in"=w48, "error in"=w47) -> ("task out"=w50:refnum<k21>, "error out"=w49:errorcluster)  [unwired: 12 in]
  n165 = call <vilib>:"DAQmx Stop Task.vi"("task/channels in"=w55, "error in"=w54) -> ("task out"=w57:refnum<k21>, "error out"=w53:errorcluster)  [unwired: 12 in]
  n166 = call <vilib>:"DAQmx Clear Task.vi"("task in"=w19, "error in"=w20) -> ()  [unwired: 13 in, 1 out]
  n167 = call <vilib>:"DAQmx Stop Task.vi"("task/channels in"=w69, "error in"=w68) -> ("task out"=w71:refnum<k21>, "error out"=w67:errorcluster)  [unwired: 12 in]
  n168 = call-poly <vilib>:"DAQmx Write.vi"("task/channels in"=w32, "data"=w30, "error in"=w25) -> ("task out"=w39:refnum<k21>, "error out"=w38:errorcluster)  [unwired: 10 in, 1 out]
  n169 = call <vilib>:"DAQmx Clear Task.vi"("task in"=w5, "error in"=w4) -> ()  [unwired: 13 in, 1 out]
  n170 = call-poly <vilib>:"DAQmx Write.vi"("task/channels in"=w36, "data"=w29, "error in"=w27) -> ("task out"=w42:refnum<k21>, "error out"=w43:errorcluster)  [unwired: 10 in, 1 out]
  n171 = call <vilib>:"DAQmx Clear Task.vi"("task in"=w50, "error in"=w49) -> ()  [unwired: 13 in, 1 out]
  n172 = call <vilib>:"DAQmx Clear Task.vi"("task in"=w57, "error in"=w53) -> ()  [unwired: 13 in, 1 out]
  n173 = call <vilib>:"DAQmx Clear Task.vi"("task in"=w71, "error in"=w67) -> ()  [unwired: 13 in, 1 out]
  n174 = call <vilib>:"DAQmx Stop Task.vi"("task/channels in"=w39, "error in"=w38) -> ("task out"=w40:refnum<k21>, "error out"=w37:errorcluster)  [unwired: 12 in]
  n175 = call <vilib>:"DAQmx Stop Task.vi"("task/channels in"=w42, "error in"=w43) -> ("task out"=w41:refnum<k21>, "error out"=w44:errorcluster)  [unwired: 12 in]
  n176 = call <vilib>:"DAQmx Clear Task.vi"("task in"=w40, "error in"=w37) -> ()  [unwired: 13 in, 1 out]
  n177 = call <vilib>:"DAQmx Clear Task.vi"("task in"=w41, "error in"=w44) -> ()  [unwired: 13 in, 1 out]
